vi "StreamTransmitAcquisitionChA.vi"() -> ()   [LabVIEW 2018]
uses:
  <resource>/objmgr/ni.dex.rc
panel:
  out "error out 2":errorcluster
  out "error out":errorcluster
  in  "stop":bool
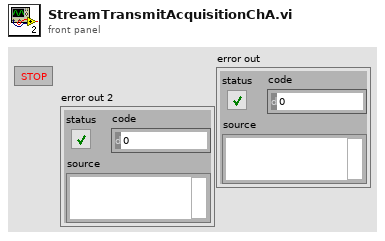
[diagram p1: front panel]
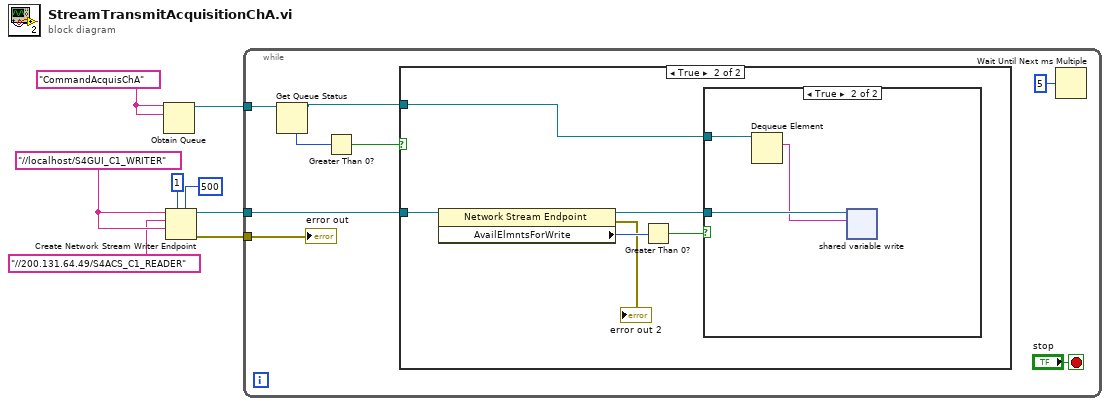
[diagram p0: block diagram]
diagram:
  w4 = "//localhost/S4GUI_C1_WRITER"
  w5 = "CommandAcquisChA"
  n1 = Obtain Queue(name (unnamed)=w5, element data type=w5) -> (queue out=w8:refnum<queue>)  [unwired: 3 in, 2 out]
  n2 = Create Network Stream Writer Endpoint(5:500 ("timeout in ms (-1)"), 7:1 ("writer buffer size"), 9:w4, 10:"//200.131.64.49/S4ACS_C1_READER", 11:w4) -> (0:w1:errorcluster, 3:w6:refnum<k21>)  [unwired: 2 in]
  n3 = while {
    tunnel: w8 -> [w15]
    tunnel: w6 -> [w11]
    tunnel: w1 -> [w9]
    stop <- "stop" stop-if-true
    n4 = Get Queue Status(queue=w15) -> (queue out=w12:refnum<queue>, # elements in queue=w14:i32)  [unwired: 2 in, 6 out]
    n5 = Greater Than 0?(x=w14) -> (x > 0?=w13:bool)
    n6 = case shown="True" w13 {
      tunnel: w12 -> [_ w22]
      tunnel: w11 -> [_ w21]
      frame False {
      }
      frame True {
        n7 = property class="Network Stream Endpoint"(reference=w21) -> (reference out=w18:refnum<k21>, error out=→"error out 2":errorcluster, "AvailElmntsForWrite"=w20:i32)  [unwired: 1 in]
        n8 = Greater Than 0?(x=w20) -> (x > 0?=w19:bool)
        n9 = case shown="True" w19 {
          tunnel: w22 -> [_ w25]
          tunnel: w18 -> [_ w24]
          frame False {
          }
          frame True {
            n10 = Dequeue Element(queue=w25) -> (element=w23:string)  [unwired: 2 in, 3 out]
            n11 = shared-variable-write(w24, w23) -> ()  [unwired: 2 in, 3 out]
          }
        }
      }
    }
    n12 = Wait Until Next ms Multiple(millisecond multiple=u32 5) -> ()  [unwired: 1 out]
    "error out" <- w9
  }
